vi "Classical Order Estimation Param Validation.vi"(6 "fs [Hz]":dbl=1.0 format="%.2f", 7 "filter type":T3, 8 "error in (no error)":errorcluster, 10 "ripple specs":T1={"passband"=0.0, "stopband"=0.0, "dB/linear? (T: dB)"=TRUE}, 11 "freq specs [Hz]":T2) -> (0 "error out":errorcluster, 2 "dup ripple specs":T1={"passband"=0.0, "stopband"=0.0, "dB/linear? (T: dB)"=TRUE}, 3 "dup freq specs [Hz]":T2)   [LabVIEW 2017, in "NI_AAL_Filter.lvlib"]
doc: "Validates the parameters for order estimation."
uses:
  <vilib>/Analysis/NI_AAL_Filter.lvlib
  <vilib>/Analysis/3filter.llb/Filter Frequence Specification (Design).ctl
  <vilib>/Analysis/3filter.llb/Filter Ripple Specification (Design).ctl
  <vilib>/Analysis/3filter.llb/Filter Passband Type.ctl
  <vilib>/Analysis/3filter.llb/Error Handlers (Multiple).vi
  <vilib>/Analysis/NI_AALBase.lvlib
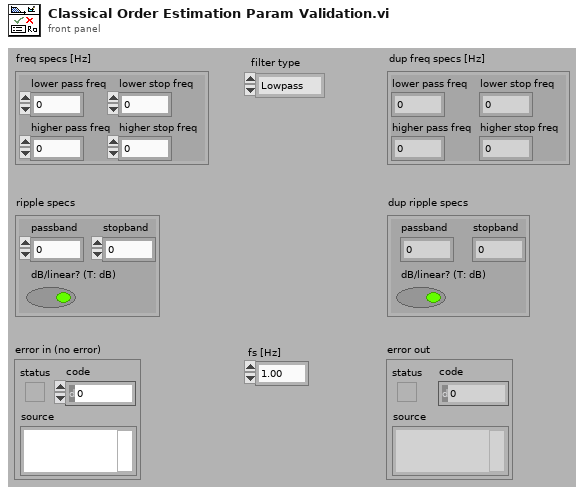
[diagram p1: front panel]
types:
  T1 = typedef "NI_AAL_Filter.lvlib/Filter Ripple Specification (Design).ctl" = cluster{"passband":dbl, "stopband":dbl, "dB/linear? (T: dB)":bool}
  T2 = typedef "NI_AAL_Filter.lvlib/Filter Frequence Specification (Design).ctl" = cluster{"lower pass freq":dbl, "lower stop freq":dbl, "higher pass freq":dbl, "higher stop freq":dbl}
  T3 = typedef "NI_AALBase.lvlib/Filter Passband Type.ctl" = enum32{"Lowpass", "Highpass", "Bandpass", "Bandstop"}
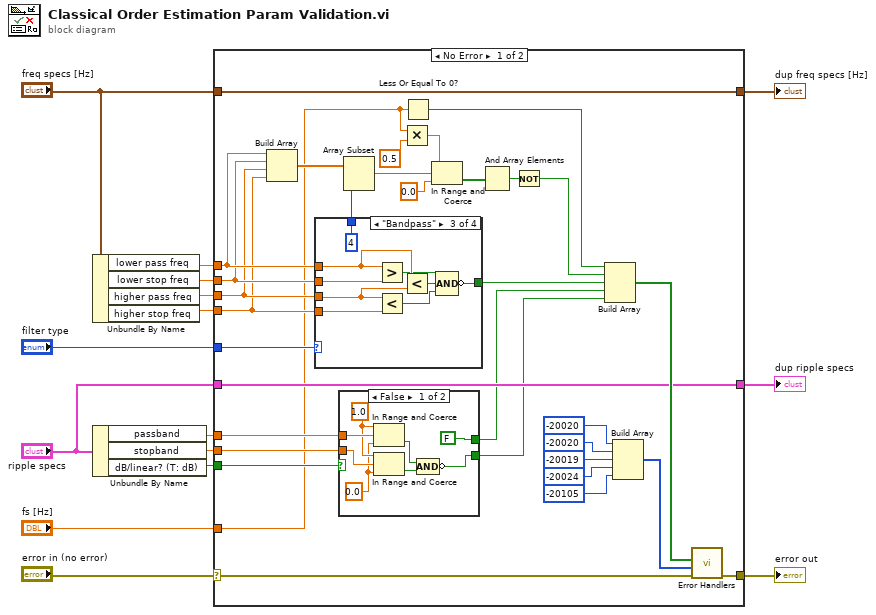
[diagram p0: block diagram]
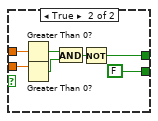
[diagram p2: hidden frame]
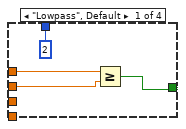
[diagram p3: hidden frame]
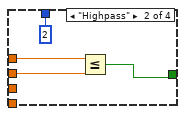
[diagram p4: hidden frame]
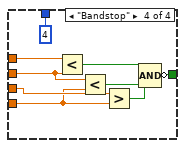
[diagram p5: hidden frame]
diagram:
  n1 = Unbundle By Name("freq specs [Hz]") -> ("lower pass freq"=w13:dbl, "lower stop freq"=w12:dbl, "higher pass freq"=w11:dbl, "higher stop freq"=w10:dbl)
  n2 = Unbundle By Name("ripple specs") -> ("passband"=w8:dbl, "stopband"=w7:dbl, "dB/linear? (T: dB)"=w9:bool)
  n3 = case shown="No Error" "error in (no error)" {
    selector: "error in (no error)" -> [w36 w90]
    tunnel: "fs [Hz]" -> [w30 _]
    tunnel: "filter type" -> [w48 _]
    tunnel: w13 -> [w42 _]
    tunnel: w12 -> [w41 _]
    tunnel: w11 -> [w40 _]
    tunnel: w10 -> [w39 _]
    tunnel: w9 -> [w45 _]
    tunnel: w8 -> [w44 _]
    tunnel: w7 -> [w43 _]
    tunnel: [w35 w90] -> w6
    tunnel: [w34 _] -> w3
    tunnel: "freq specs [Hz]" -> [w34 _]
    tunnel: "ripple specs" -> [w33 _]
    tunnel: [w33 _] -> w1
    frame No Error {
      n4 = Build Array(w42, w41, w40, w39) -> (w32:dbl[])
      n5 = case shown="\"Bandpass\"" w48 {
        tunnel: w42 -> [w67 w71 w78 w89]
        tunnel: w41 -> [w66 w70 w80 w88]
        tunnel: w40 -> [_ _ w77 w87]
        tunnel: w39 -> [_ _ w79 w81]
        tunnel: [w65 w69 w73 w83] -> w47
        tunnel: [2 2 4 4] -> w31
        frame "Lowpass", Default {
          n6 = Greater Or Equal?(x=w67, y=w66) -> (x >= y?=w65:bool)
        }
        frame "Highpass" {
          n7 = Less Or Equal?(x=w71, y=w70) -> (x <= y?=w69:bool)
        }
        frame "Bandpass" {
          n8 = Greater?(x=w78, y=w80) -> (0:w76:bool)
          n9 = Less?(x=w77, y=w79) -> (x < y?=w74:bool)
          n10 = Less?(x=w78, y=w77) -> (x < y?=w75:bool)
          n11 = Compound Arithmetic op=AND(w76, w75, w74) -> (invert w73:bool)
        }
        frame "Bandstop" {
          n12 = Less?(x=w89, y=w88) -> (x < y?=w86:bool)
          n13 = Less?(x=w88, y=w81) -> (x < y?=w85:bool)
          n14 = Greater?(x=w87, y=w81) -> (0:w84:bool)
          n15 = Compound Arithmetic op=AND(w86, w85, w84) -> (invert w83:bool)
        }
      }
      n16 = case shown="False" w45 {
        tunnel: w44 -> [w55 w61]
        tunnel: w43 -> [w56 w63]
        tunnel: [w50 FALSE] -> w17
        tunnel: [FALSE w57] -> w19
        frame False {
          w53 = 0.0 ("lower limit")
          w54 = 1.0 ("y")
          n17 = In Range and Coerce(upper limit=w54, x=w55, lower limit=w53) -> (In Range?=w52:bool)  [unwired: 1 out]
          n18 = In Range and Coerce(upper limit=w54, x=w56, lower limit=w53) -> (In Range?=w51:bool)  [unwired: 1 out]
          n19 = Compound Arithmetic op=AND(w52, w51) -> (invert w50:bool)
        }
        frame True {
          n20 = Greater Than 0?(x=w61) -> (x > 0?=w60:bool)
          n21 = Greater Than 0?(x=w63) -> (x > 0?=w59:bool)
          n22 = And(x=w60, y=w59) -> (x .and. y?=w58:bool)
          n23 = Not(x=w58) -> (.not. x?=w57:bool)
        }
      }
      n24 = Array Subset(array=w32, length=w31) -> (w28:dbl[])  [unwired: 1 in]
      n25 = Multiply(x=w30, y=0.5) -> (x*y=w21:dbl)
      n26 = Less Or Equal To 0?(x=w30) -> (x <= 0?=w22:bool)
      n27 = In Range and Coerce(upper limit=w21, x=w28, lower limit=0.0) -> (In Range?=w27:bool[])  [unwired: 1 out]
      n28 = And Array Elements(Boolean array=w27) -> (logical AND=w26:bool)
      n29 = Not(x=w26) -> (.not. x?=w25:bool)
      n30 = Build Array(w22, w25, w47, w19, w17) -> (w37:bool[])
      n31 = Build Array(-20020 ("ERR_FS_LE_ZERO"), -20020 ("ERR_FREQ_RANGE_WRONG"), -20019 ("ERR_FREQ_SEQ_WRONG"), -20024 ("ERR_FREQ_SEQ_WRONG"), -20105 ("ERR_RIPPLE_RANGE_WRONG")) -> (w38:i32[])
      n32 = call-poly <vilib>:"Error Handlers.vi"("error in (no error)"=w36, "error sources"=w38, "condition failed?"=w37) -> ("error out"=w35:errorcluster)  [unwired: 8 out]
    }
    frame Error {
    }
  }
  "error out" <- w6
  "dup freq specs [Hz]" <- w3
  "dup ripple specs" <- w1
